vi "DMM-261 Mux Group.vi"() -> ()   [LabVIEW 8.6]
uses:
  <libdir>/resource/objmgr/UeiDaq.rc
  <vilib>/UeiDaq/UeiDaqConfigureTimingForSimpleIO.vi
  <vilib>/UeiDaq/UeiDaqReadOneScaledScan.vi
panel:
  in  "Auto-Range":i32(ring) items=["Disable", "Enable"]
  in  "Measurement Mode":i32(ring) items=["Calibrated DC Voltage", "Averaged NPLC DC Voltage", "RMS AC Voltage", "Averaged RMS AC Voltage", "Min AC Peak Voltage", "Max AC Peak Voltage", "Frequency AC Voltage", "Calibrated DC Current", "Averaged NPLC DC Current", "RMS AC Current", "Averaged RMS AC Current", "Min AC Peak Current", "Max AC Peak Current", "Frequency AC Current", "Two-wire Resistance", "Four-wire Resistance", "Guardian DC Voltage Vref", "Guardian DC Current Vref", "Guardian DC Current", "Guardian AC Current", "Guardian Voltage 0", "Guardian Voltage 1", "Guardian Voltage 2", "Guardian Voltage 3", "Guardian Temperature"]
  in  "Refresh rate (ms)":u32
  in  "Store Config":bool
  in  "Mux Relay Select":i32(ring) items=["Disable", "A Relay", "B Relay", "AB Relays"]
  in  "Mux Channel Number":i32
  in  "Mux Device Number":i32
  in  "Number of Mux Devices":i32
  in  "timeout (ms)":u32
  in  "Range":dbl
  in  "Resource":string
  out "Total scans acquired":u32
  out "Waveform Chart":dbl[][](graph)
  in  "stop":bool
  # "DMM-261 Mux Group Acquisition"
  # "DMM Configuration"
  # "DMM-261 configuration\ncan only be modified\nBEFORE the session\nis started"
  # "Total number of Mux devices\nconnected to the DMM-261"
  # "MUX Configuration"
  # "Mux device number in the IOM\nto connect to the DMM-261"
  # "Mux relay select. AB is only\navailable when using 4-wire\nResistance Measurement"
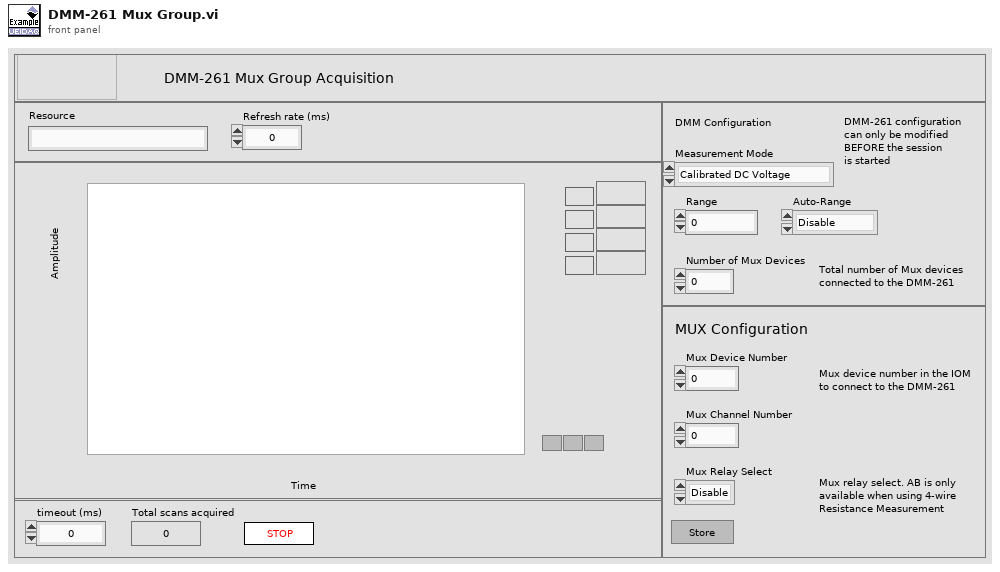
[diagram p1: front panel]
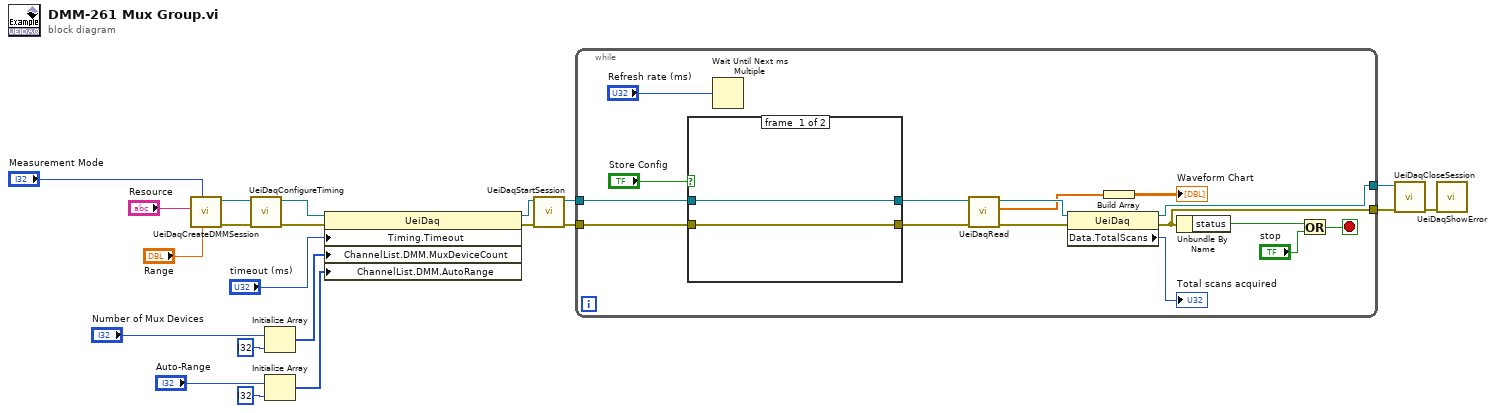
[diagram p0: block diagram]
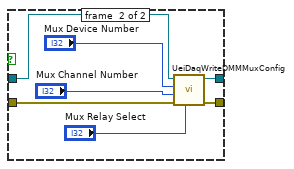
[diagram p2: hidden frame]
diagram:
  n1 = call <vilib>:"UeiDaqCreateDMMSession.vi"("Range"="Range", "Measurement Mode"="Measurement Mode", "Resource"="Resource") -> ("error out"=w14:errorcluster, "UeiDaq Refnum Out"=w13:refnum<k20>)  [unwired: 7 in]
  n2 = call-poly <vilib>:"UeiDaqConfigureTiming.vi"("error in (no error)"=w14, "UeiDaq Refnum In"=w13) -> ("error out"=w18:errorcluster, "UeiDaq Refnum Out"=w17:refnum<k20>)  [unwired: 1 in, 7 out]
  n3 = Initialize Array("Number of Mux Devices", i32 ? ("dimension size")) -> (w5:i32[])
  n4 = Initialize Array("Auto-Range", i32 ? ("dimension size")) -> (w1:i32[])
  n5 = property class="UeiDaq"(reference=w17, error in=w18, "Timing.Timeout"="timeout (ms)", "ChannelList.DMM.MuxDeviceCount"=w5, "ChannelList.DMM.AutoRange"=w1) -> (reference out=w11:refnum<k20>, error out=w10:errorcluster)
  n6 = call <vilib>:"UeiDaqStartSession.vi"("error in (no error)"=w10, "UeiDaq Refnum In"=w11) -> ("error out"=w9:errorcluster, "UeiDaq Refnum Out"=w8:refnum<k20>)  [unwired: 8 in]
  n7 = while {
    tunnel: [w36] -> w19
    tunnel: [w35] -> w20
    tunnel: w9 -> [w26]
    tunnel: w8 -> [w27]
    stop <- w37 stop-if-true
    n8 = case shown="True" "Store Config" {
      tunnel: w27 -> [w39 w46]
      tunnel: w26 -> [w38 w45]
      tunnel: [w39 w44] -> w25
      tunnel: [w38 w43] -> w24
      frame #0 {
      }
      frame #1 {
        n9 = call "UeiDaqWriteDMMMuxConfig.vi"("Mux Relay Select"="Mux Relay Select", "error in (no error)"=w45, "Mux Channel Number"="Mux Channel Number", "Mux Device Number"="Mux Device Number", "UeiDaq Refnum In"=w46) -> ("error out"=w43:errorcluster, "UeiDaq Refnum Out"=w44:refnum<k20>)  [unwired: 5 in]
      }
    }
    n10 = Wait Until Next ms Multiple(millisecond multiple="Refresh rate (ms)") -> ()  [unwired: 1 out]
    n11 = call-poly <vilib>:"UeiDaqRead.vi"("error in (no error)"=w24, "UeiDaq Refnum In"=w25) -> ("error out"=w30:errorcluster, "Scaled Data"=w29:dbl[], "UeiDaq Refnum Out"=w31:refnum<k20>)  [unwired: 7 out]
    n12 = property class="UeiDaq"(reference=w31, error in=w30) -> (reference out=w35:refnum<k20>, error out=w36:errorcluster, "Data.TotalScans"=→"Total scans acquired":u32)
    n13 = Build Array(w29) -> (→"Waveform Chart":dbl[][])
    n14 = Unbundle By Name(w36) -> ("status"=w32:bool)
    n15 = Or(x=w32, y="stop") -> (x .or. y?=w37:bool)
  }
  n16 = call <vilib>:"UeiDaqCloseSession.vi"("error in (no error)"=w19, "UeiDaq Refnum In"=w20) -> ("error out"=w21:errorcluster)  [unwired: 1 in, 8 out]
  n17 = call <vilib>:"UeiDaqShowError.vi"("error in (no error)"=w21) -> ()  [unwired: 2 in, 9 out]
